vi "Process Joystick Axis Motion Event.vi"(6 "Value":i16, 9 "Axis":u8, 10 "Player":T1) -> ()   [LabVIEW 2021, in "Main Controller Actor.lvclass"]
uses:
  Main Controller Actor.lvclass
  Ship/Ship.lvclass
  C:/dev/LabVIEW/LabMelee/Source/Application Specific/Element/Element.lvclass
  Ship/Ship.lvclass/Ship.ctl
  Control State/Control State.lvclass/Control State.ctl
  Main Controller Actor.lvclass/Main Controller Actor.ctl
  C:/dev/LabVIEW/LabMelee/Source/Application Specific/Ship/Ship.lvclass
  Control State/Control State.lvclass
  Globals.vi
  Player.ctl
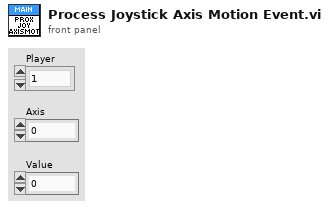
[diagram p1: front panel]
types:
  T1 = typedef "Main Controller Actor.lvclass/Player.ctl" = enum16{"1", "2"}
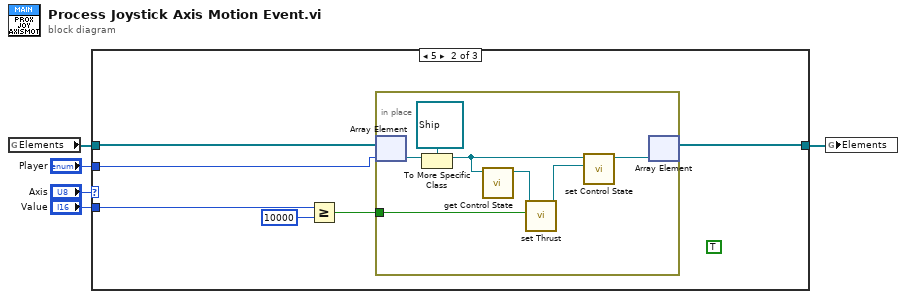
[diagram p0: block diagram]
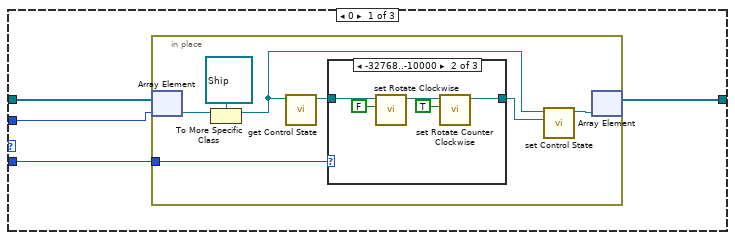
[diagram p2: hidden frame]
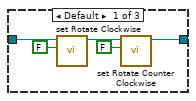
[diagram p3: hidden frame]
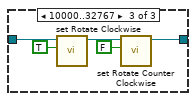
[diagram p4: hidden frame]
diagram:
  n1 = global read "Globals.vi" "Elements"() -> (w2:refnum<class "Element.lvclass">[])
  n2 = case shown="5" "Axis" {
    tunnel: "Value" -> [w9 w37 _]
    tunnel: "Player" -> [w8 w36 _]
    tunnel: w2 -> [w7 w33 w45]
    tunnel: [w6 w32 w45] -> w1
    frame 0 {
      n3 = in-place {
        in-place-border: w9 -> [w16]
        n4 = in-place-array #1(w7, w8) -> (w11:refnum<class "Element.lvclass">)
        n5 = To More Specific Class(target class=refnum<class "Ship.lvclass"> refnum ("Ship in"), reference=w11) -> (specific class reference=w10:refnum<class "Ship.lvclass">)  [unwired: 1 in, 1 out]
        n6 = call "get Control State.vi"("Ship in"=w10) -> ("Control State"=w15:refnum<class "Control State.lvclass">)  [unwired: 10 in]
        n7 = case shown="-32768..-10000" w16 {
          tunnel: w15 -> [w21 w26 w31]
          tunnel: [w19 w24 w29] -> w14
          frame Default {
            n8 = call "set Rotate Clockwise.vi"("Rotate Clockwise"=FALSE, "Control State in"=w21) -> ("Control State out"=w20:refnum<class "Control State.lvclass">)  [unwired: 9 in]
            n9 = call "set Rotate Counter Clockwise.vi"("Rotate Counter Clockwise"=FALSE, "Control State in"=w20) -> ("Control State out"=w19:refnum<class "Control State.lvclass">)  [unwired: 9 in]
          }
          frame -32768..-10000 {
            n10 = call "set Rotate Clockwise.vi"("Rotate Clockwise"=FALSE, "Control State in"=w26) -> ("Control State out"=w25:refnum<class "Control State.lvclass">)  [unwired: 9 in]
            n11 = call "set Rotate Counter Clockwise.vi"("Rotate Counter Clockwise"=TRUE, "Control State in"=w25) -> ("Control State out"=w24:refnum<class "Control State.lvclass">)  [unwired: 9 in]
          }
          frame 10000..32767 {
            n12 = call "set Rotate Clockwise.vi"("Rotate Clockwise"=TRUE, "Control State in"=w31) -> ("Control State out"=w30:refnum<class "Control State.lvclass">)  [unwired: 9 in]
            n13 = call "set Rotate Counter Clockwise.vi"("Rotate Counter Clockwise"=FALSE, "Control State in"=w30) -> ("Control State out"=w29:refnum<class "Control State.lvclass">)  [unwired: 9 in]
          }
        }
        n14 = call-dynamic "set Control State.vi"("Control State"=w14, "Ship in"=w10) -> ("Ship out"=w13:refnum<class "Ship.lvclass">)  [unwired: 9 in]
        n15 = in-place-array #1(w13) -> (w6:refnum<class "Element.lvclass">[])  [unwired: 1 out]
      }
    }
    frame 5 {
      (unwired) TRUE
      n16 = Greater Or Equal?(x=w37, y=i16 10000) -> (x >= y?=w34:bool)
      n17 = in-place {
        in-place-border: w34 -> [w44]
        n18 = in-place-array #2(w33, w36) -> (w40:refnum<class "Element.lvclass">)
        n19 = To More Specific Class(target class=refnum<class "Ship.lvclass"> refnum ("Ship in"), reference=w40) -> (specific class reference=w38:refnum<class "Ship.lvclass">)  [unwired: 1 in, 1 out]
        n20 = call "get Control State.vi"("Ship in"=w38) -> ("Control State"=w43:refnum<class "Control State.lvclass">)  [unwired: 10 in]
        n21 = call "set Thrust.vi"("Thrust"=w44, "Control State in"=w43) -> ("Control State out"=w42:refnum<class "Control State.lvclass">)  [unwired: 9 in]
        n22 = call-dynamic "set Control State.vi"("Control State"=w42, "Ship in"=w38) -> ("Ship out"=w41:refnum<class "Ship.lvclass">)  [unwired: 9 in]
        n23 = in-place-array #2(w41) -> (w32:refnum<class "Element.lvclass">[])  [unwired: 1 out]
      }
    }
    frame Default {
    }
  }
  n24 = global write "Globals.vi" "Elements"(w1) -> ()
